vi "Priority Queue Test.vi"() -> (3 "Pass?":bool)   [LabVIEW 2014]
uses:
  <vilib>/ActorFramework/Stop Msg/Stop Msg.lvclass
  <vilib>/ActorFramework/Message Enqueuer/Message Priority.ctl
  <vilib>/ActorFramework/Message Queue/Message Queue.lvclass/Message Queue.ctl
  Increment Msg/Increment Msg.lvclass/Increment Msg.ctl
  <vilib>/ActorFramework/Message Enqueuer/Message Enqueuer.lvclass/Message Enqueuer.ctl
  <vilib>/ActorFramework/Stop Msg/Stop Msg.lvclass/Stop Msg.ctl
  <vilib>/ActorFramework/Message Dequeuer/Message Dequeuer.lvclass/Message Dequeuer.ctl
  Increment Msg/Increment Msg.lvclass
  <vilib>/ActorFramework/Message Enqueuer/Enqueue.vi
  <vilib>/ActorFramework/Message Enqueuer/Enqueue Critical.vi
  <vilib>/ActorFramework/Message Priority Queue/Priority Enqueue.vi
  <vilib>/ActorFramework/Message Priority Queue/Priority Dequeue.vi
  <vilib>/ActorFramework/Message Enqueuer/Message Enqueuer.lvclass
  <vilib>/ActorFramework/Message Queue/Message Queue.lvclass
  <vilib>/ActorFramework/Message Dequeuer/Message Dequeuer.lvclass
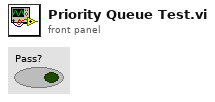
[diagram p1: front panel]
types:
  T1 = typedef "Actor Framework.lvlib/Message Enqueuer.lvclass/Message Priority.ctl" = enum16{"Low", "Normal", "High"}
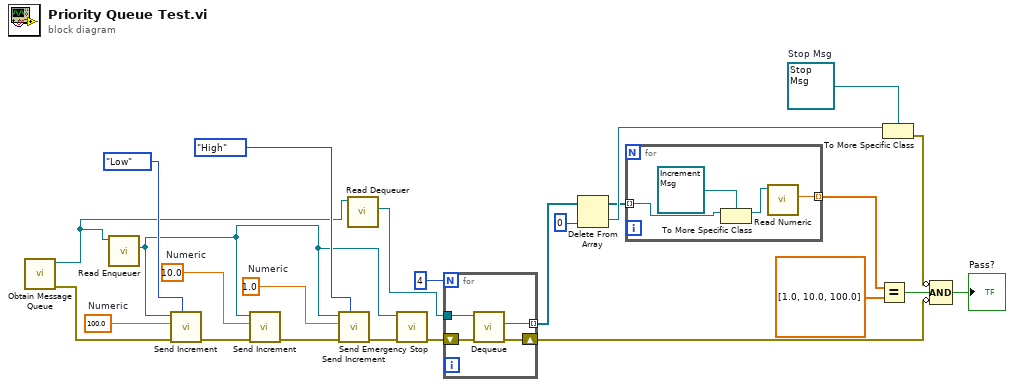
[diagram p0: block diagram]
diagram:
  w15 = refnum<class "Stop Msg.lvclass"> refnum  # Stop Msg
  w21 = 1.0  # Numeric
  w23 = 10.0  # Numeric
  w25 = 100.0  # Numeric
  n1 = call <vilib>:"Obtain Message Queue.vi"() -> ("error out"=w4:errorcluster, "Message Queue"=w2:refnum<class "Message Queue.lvclass">)  [unwired: 10 in]
  n2 = call <vilib>:"Read Enqueuer.vi"("Message Queue"=w2) -> ("Message Enqueuer"=w3:refnum<class "Message Enqueuer.lvclass">)  [unwired: 10 in]
  n3 = call "Send Increment.vi"("Message Priority"=Message_Priority."Low", "error in (no error)"=w4, "Numeric"=w25, "Actor Framework.lvlib:Send Queue"=w3) -> ("error out"=w24:errorcluster)  [unwired: 7 in]
  n4 = call "Send Increment.vi"("error in (no error)"=w24, "Numeric"=w23, "Actor Framework.lvlib:Send Queue"=w3) -> ("error out"=w22:errorcluster)  [unwired: 8 in]
  n5 = call "Send Increment.vi"("Message Priority"=Message_Priority."High", "error in (no error)"=w22, "Numeric"=w21, "Actor Framework.lvlib:Send Queue"=w3) -> ("error out"=w20:errorcluster)  [unwired: 7 in]
  n6 = call <vilib>:"Read Dequeuer.vi"("Message Queue"=w2) -> ("Message Dequeuer"=w1:refnum<class "Message Dequeuer.lvclass">)  [unwired: 10 in]
  n7 = call <vilib>:"Send Emergency Stop.vi"("error in (no error)"=w20, "Message Enqueuer"=w3) -> ("error out"=w7:errorcluster)  [unwired: 9 in]
  n8 = for {
    N: 4 -> [_]
    tunnel: w1 -> [w27]
    tunnel: [w26] -> w18 mode=indexing
    shift-right: [w28] -> w8
    shift-left: w7 -> [w29]
    n9 = call <vilib>:"Dequeue.vi"("error in (no error)"=w29, "Message Dequeuer in"=w27) -> ("error out"=w28:errorcluster, "Message"=w26:refnum<class "Message.lvclass">)  [unwired: 5 in, 3 out]
  }
  n10 = Delete From Array(array=w18, index=0) -> (deleted portion=w16:refnum<class "Message.lvclass">, array with subset deleted=w13:refnum<class "Message.lvclass">[])  [unwired: 1 in]
  n11 = for {
    tunnel: w13 -> [w33] mode=indexing
    tunnel: [w30] -> w12 mode=indexing
    n12 = To More Specific Class(target class=refnum<class "Increment Msg.lvclass"> refnum ("Object"), reference=w33) -> (specific class reference=w31:refnum<class "Increment Msg.lvclass">)  [unwired: 1 in, 1 out]
    n13 = call "Read Numeric.vi"("Increment Msg in"=w31) -> ("Numeric"=w30:dbl)  [unwired: 9 in, 1 out]
  }
  n14 = Equal?(x=w12, y=dbl[] [1.0, 10.0, 100.0]) -> (x = y?=w10:bool)
  n15 = To More Specific Class(target class=w15, reference=w16) -> (error out=w14:errorcluster)  [unwired: 1 in, 1 out]
  n16 = Compound Arithmetic op=AND(invert w14, w10, invert w8) -> (→"Pass?":bool)
